vi "Configure Arbitrary Waveform.vi"(5 "Select Channel (1:Channel 1)":i32(ring)=1 items=["Channel 1"=1, "Channel 2"=2], 6 "DC Offset (0.00 V)":dbl min=-10.0 max=10.0, 7 "Amplitude (1.0 Vpp)":dbl=1.0 min=0.001 max=20.0 step=1.0 format="%#.3f", 8 "error in (no error)":errorcluster, 9 "Phase (0.0 degrees)":dbl=0.002 min=-360.0 max=360.0 format="%#.1g", 10 "Frequency (1000 Hz)":dbl=1000.0 min=1e-06 max=160000000.0 step=1.0 format="%#.6g", 11 "VISA resource name":refnum<visa-resource-name>) -> (0 "error out":errorcluster, 3 "VISA resource name out":refnum<visa-resource-name>)   [LabVIEW 2015]
doc: "Sets the waveform parameters for an arbitrary waveform. This VI should be called after <b>Create Arbitrary Waveform.vi</b> (for user defined arbitrary waveform) and <b>Select Arbitrary Waveform.vi</b>"
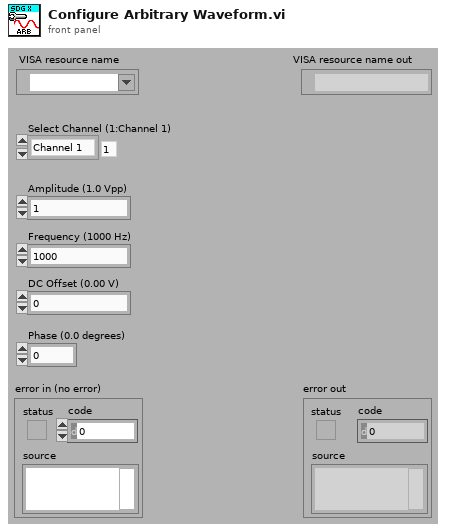
[diagram p1: front panel]
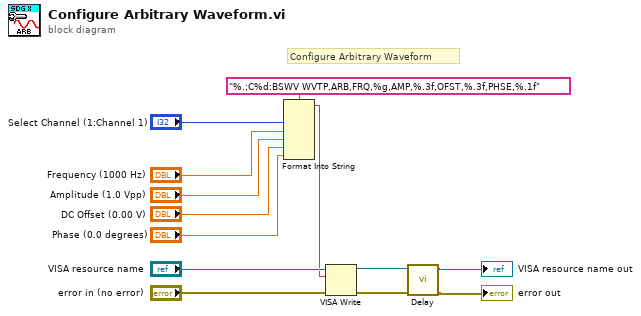
[diagram p0: block diagram]
diagram:
  # "Configure Arbitrary Waveform"
  n1 = Format Into String(format string="%.;C%d:BSWV WVTP,ARB,FRQ,%g,AMP,%.3f,OFST,%.3f,PHSE,%.1f", "Select Channel (1:Channel 1)", "Frequency (1000 Hz)", "Amplitude (1.0 Vpp)", "DC Offset (0.00 V)", "Phase (0.0 degrees)") -> (resulting string=w10:string)  [unwired: 2 in, 1 out]
  n2 = VISA Write(VISA resource name="VISA resource name", write buffer=w10, error in (no error)="error in (no error)") -> (VISA resource name out=w9:refnum<visa-resource-name>, error out=w8:errorcluster)  [unwired: 1 out]
  n3 = call <instrlib>:"Delay.vi"("error in (no error)"=w8, "VISA resource name"=w9) -> ("error out"=→"error out":errorcluster, "VISA resource name out"=→"VISA resource name out":refnum<visa-resource-name>)  [unwired: 8 in]
